vi "LABVIWE_SORTING_WHILE_LOOP.vi"() -> ()   [LabVIEW 2020]
panel:
  out "sorted array":dbl[](array[numeric])
  out "Array":dbl[](array[numeric])
  in  "array":dbl[](array[numeric])
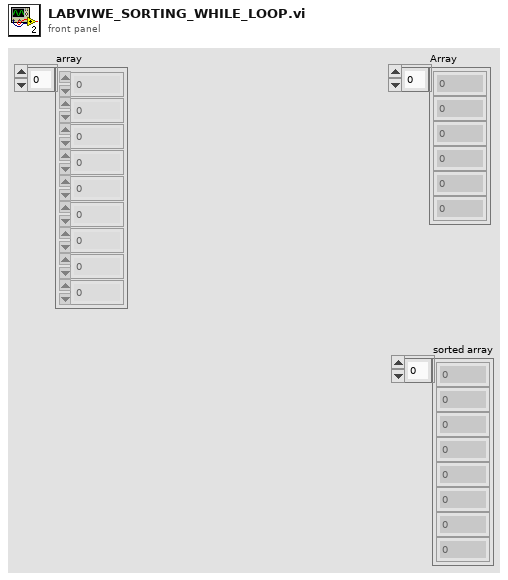
[diagram p1: front panel]
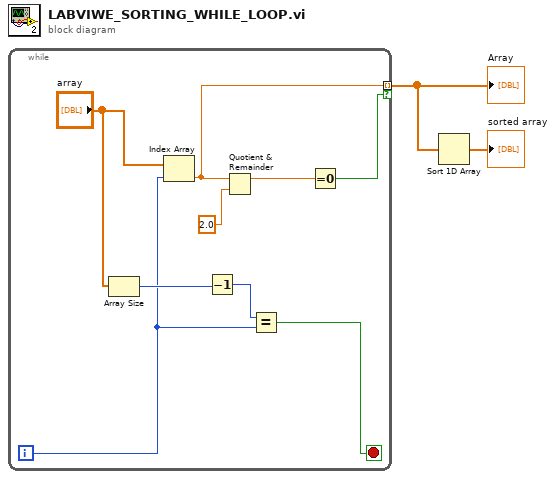
[diagram p0: block diagram]
diagram:
  n1 = while {
    tunnel: [w4] -> w2 mode=indexing if=w10
    i -> [w6]
    stop <- w5 stop-if-true
    n2 = Array Size(array="array") -> (size(s)=w8:i32)
    n3 = Index Array "Index Array"(array="array", index=w6) -> (element=w4:dbl)
    n4 = Decrement(x=w8) -> (x-1=w7:i32)
    n5 = Quotient & Remainder(x=w4, y=2.0) -> (x-y*floor(x/y)=w11:dbl)  [unwired: 1 out]
    n6 = Equal?(x=w7, y=w6) -> (x = y?=w5:bool)
    n7 = Equal To 0?(x=w11) -> (x = 0?=w10:bool)
  }
  "Array" <- w2
  n8 = Sort 1D Array(array=w2) -> (sorted array=→"sorted array":dbl[])
